vi "Read Reports.vi"(8 "error in (no error)":errorcluster, 11 "Report Action in":refnum<class "Report Action.lvclass">) -> (0 "error out":errorcluster, 2 "Reports":refnum<class "Report Data.lvclass">[](array[class]), 3 "Report Action out":refnum<class "Report Action.lvclass">)   [LabVIEW 2020, in "ProjectBuilder.lvlib" / "Report Action.lvclass"]
uses:
  Report Action.lvclass
  Data/Report Data/Report Data.lvclass
  Report Action.lvclass/Report Action.ctl
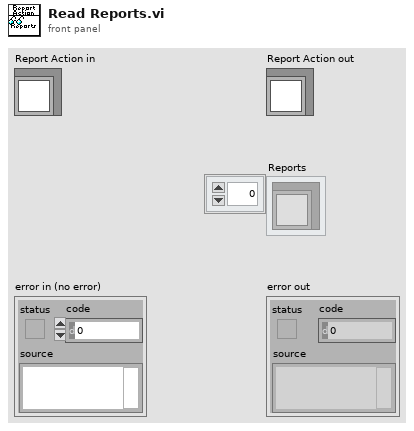
[diagram p1: front panel]
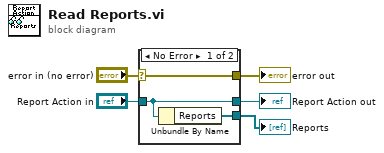
[diagram p0: block diagram]
diagram:
  n1 = case shown="No Error" "error in (no error)" {
    selector: "error in (no error)" -> [w8 w9]
    tunnel: [w8 w9] -> w4
    tunnel: [w7 w10] -> w2
    tunnel: "Report Action in" -> [w7 w10]
    tunnel: [w6 _] -> w1
    frame No Error {
      n2 = Unbundle By Name(w7) -> ("Reports"=w6:refnum<class "Report Data.lvclass">[])
    }
    frame Error {
    }
  }
  "error out" <- w4
  "Report Action out" <- w2
  "Reports" <- w1
